vi "ListConfigurations.vi"(8 "ErrorIn":errorcluster, 11 "ObjectIn":refnum<class "IApplicationConfiguration.lvclass">) -> (0 "ErrorOut":errorcluster, 2 "Identification":string[](array[string]), 3 "ObjectOut":refnum<class "IApplicationConfiguration.lvclass">)   [LabVIEW 2021, in "IApplicationConfiguration.lvclass"]
uses:
  IApplicationConfiguration.lvclass
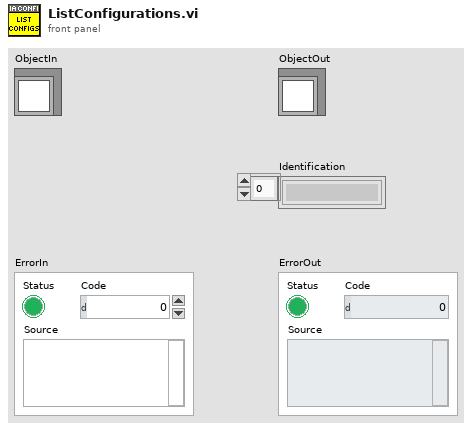
[diagram p1: front panel]
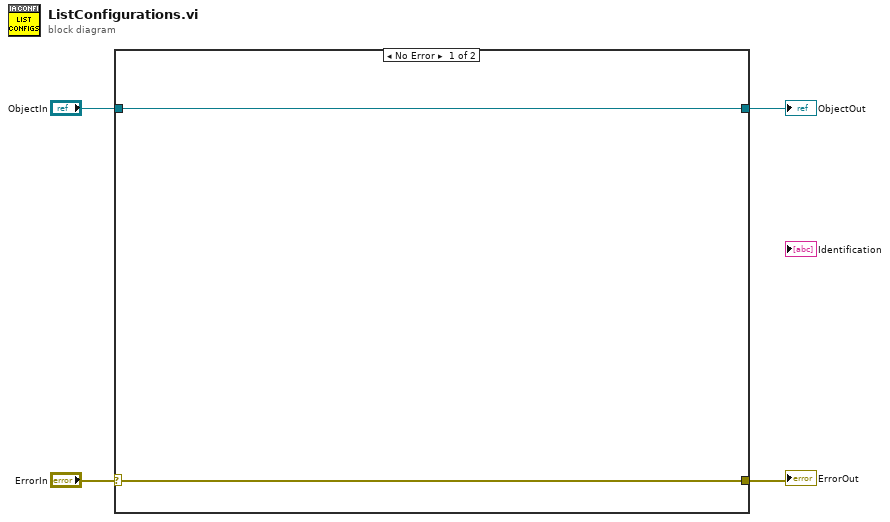
[diagram p0: block diagram]
diagram:
  n1 = case shown="No Error" "ErrorIn" {
    selector: "ErrorIn" -> [w6 w8]
    tunnel: [w6 w8] -> w3
    tunnel: [w5 w7] -> w1
    tunnel: "ObjectIn" -> [w5 w7]
    frame No Error {
    }
    frame Error {
    }
  }
  "ErrorOut" <- w3
  "ObjectOut" <- w1
